vi "Init Panels.vi"(8 "error in (no error)":errorcluster, 11 "TouchControl in":refnum<class "TouchControl.lvclass">) -> (0 "error out":errorcluster, 3 "TouchControl out":refnum<class "TouchControl.lvclass">)   [LabVIEW 2022 SP3, in "TouchControl.lvlib" / "TouchControl.lvclass"]
uses:
  TouchControl.lvclass
  LightsPanel/LightsPanel.lvclass
  C:/Program Files (x86)/National Instruments/LabVIEW 2022/vi.lib/IlluminatedG/IG OOPanel/OOPanel/Panel/Panel.lvclass
  AudioMonPanel/AudioMonPanel.lvclass
  TouchControl.lvclass/TouchControl.ctl
  MuxPanel/MuxPanel.lvclass
  <vilib>/IlluminatedG/IG OOPanel/OOPanel/Manager/Manager.lvclass
  TouchControl.lvlib
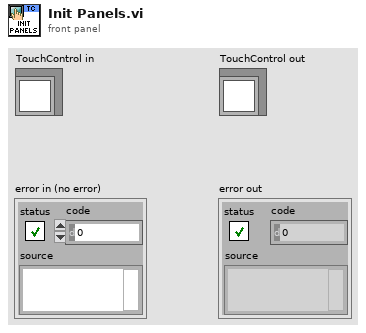
[diagram p1: front panel]
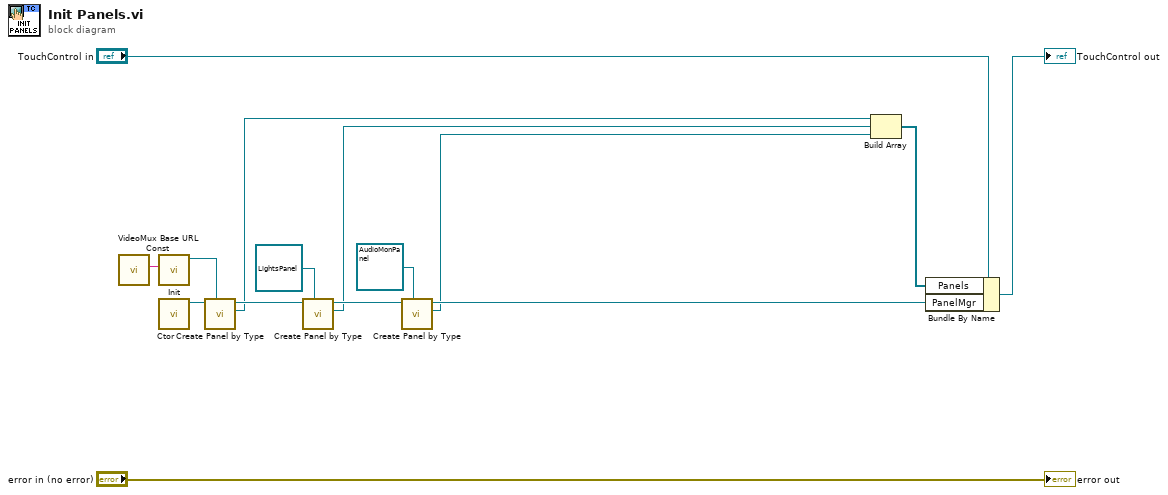
[diagram p0: block diagram]
diagram:
  n1 = call "VideoMux Base URL Const.vi"() -> ("VideoMux Base URL"=w1:string)  [unwired: 11 in]
  n2 = call "Init.vi"("VideoMux Base URL"=w1) -> ("MuxPanel out"=w2:refnum<class "MuxPanel.lvclass">)  [unwired: 9 in, 1 out]
  n3 = call <vilib>:"Ctor.vi"() -> ("Manager out"=w13:refnum<class "Manager.lvclass">)  [unwired: 10 in, 1 out]
  n4 = call <vilib>:"Create Panel by Type.vi"("Panel Type"=w2, "Manager in"=w13) -> ("Panel"=w10:refnum<class "MuxPanel.lvclass">, "Manager out"=w11:refnum<class "Manager.lvclass">)  [unwired: 7 in, 1 out]
  n5 = call <vilib>:"Create Panel by Type.vi"("Panel Type"=refnum<class "LightsPanel.lvclass"> refnum ("TouchControl.lvlib:LightsPanel.lvclass"), "Manager in"=w11) -> ("Panel"=w6:refnum<class "LightsPanel.lvclass">, "Manager out"=w8:refnum<class "Manager.lvclass">)  [unwired: 7 in, 1 out]
  n6 = call <vilib>:"Create Panel by Type.vi"("Panel Type"=refnum<class "AudioMonPanel.lvclass"> refnum ("TouchControl.lvlib:AudioMonPanel.lvclass"), "Manager in"=w8) -> ("Panel"=w3:refnum<class "AudioMonPanel.lvclass">, "Manager out"=w5:refnum<class "Manager.lvclass">)  [unwired: 7 in, 1 out]
  n7 = Build Array(w10, w6, w3) -> (w9:refnum<class "Panel.lvclass">[])
  n8 = Bundle By Name(cluster="TouchControl in", "Panels"=w9, "PanelMgr"=w5) -> (→"TouchControl out":refnum<class "TouchControl.lvclass">)
  "error out" <- "error in (no error)"
